vi "Do.vi"(8 "error in (no error)":errorcluster, 10 "Actor in":refnum<class "Actor.lvclass">, 11 "Concrete Tool Buttons Pressed Msg in":refnum<class "Concrete Tool Buttons Pressed Msg.lvclass">) -> (0 "error out":errorcluster, 2 "Actor out":refnum<class "Actor.lvclass">)   [LabVIEW 2020, in "Map View.lvlib" / "Concrete Tool Buttons Pressed Msg.lvclass"]
doc: "(<B>Filename</B>: Actor Framework.lvlib:Message.lvclass:Do.vi)\n\nDefines what a message does when it is received by an actor. Generally, a message instructs an actor to invoke one of its methods.\n\nBy default, this method does nothing. A child class must override it to define behavior. Create a child class by using the Actor Framework Message Maker dialog box."
uses:
  Concrete Tool Buttons Pressed Msg.lvclass
  E:/Project/Labview-Projects/Completed projects/Map Editor/Views/Tools View/Tools View Messages/Abstract Tool Buttons Pressed Msg/Abstract Tool Buttons Pressed Msg.lvclass
  <vilib>/ActorFramework/Actor/Actor.lvclass
  Map View/Map View.lvclass
  C:/Program Files/National Instruments/LabVIEW 2020/vi.lib/ActorFramework/Actor/Actor.lvclass
  Tools View/Tools View Messages/Abstract Tool Buttons Pressed Msg/Abstract Tool Buttons Pressed Msg.lvclass
panel:
  # "NOTICE -- YOU MUST LEAVE THIS NOTICE IN PLACE.\n\nCopyright (c) 2017, LIANG LIU Shawn.Liu.cn@gmail.com\nAll rights reserved.\n\nRedistribution and use in source and binary forms, with or without modification, are permitted provided that the following conditions are met:\n-Redistributions of source code must retain the above copyright notice, this list of conditions and the following disclaimer.\n-Redistributions in binary form must reproduce the above copyright notice, this list of conditions and the following disclaimer in the documentation and/or other materials provided with the distribution.\n-Neither the name of the eLp nor the names of its contributors may be used to endorse or promote products derived from this software without specific prior written permission.\n\nTHIS SOFTWARE IS PROVIDED BY THE COPYRIGHT HOLDERS AND CONTRIBUTORS \"AS IS\" AND ANY EXPRESS OR IMPLIED WARRANTIES, INCLUDING, BUT NOT LIMITED TO, THE IMPLIED WARRANTIES OF MERCHANTABILITY AND FITNESS FOR A PARTICULAR PURPOSE ARE DISCLAIMED. IN NO EVENT SHALL THE COPYRIGHT HOLDER OR CONTRIBUTORS BE LIABLE FOR ANY DIRECT, INDIRECT, INCIDENTAL, SPECIAL, EXEMPLARY, OR CONSEQUENTIAL DAMAGES (INCLUDING, BUT NOT LIMITED TO, PROCUREMENT OF SUBSTITUTE GOODS OR SERVICES; LOSS OF USE, DATA, OR PROFITS; OR BUSINESS INTERRUPTION) HOWEVER CAUSED AND ON ANY THEORY OF LIABILITY, WHETHER IN CONTRACT, STRICT LIABILITY, OR TORT (INCLUDING NEGLIGENCE OR OTHERWISE) ARISING IN ANY WAY OUT OF THE USE OF THIS SOFTWARE, EVEN IF ADVISED OF THE POSSIBILITY OF SUCH DAMAGE."
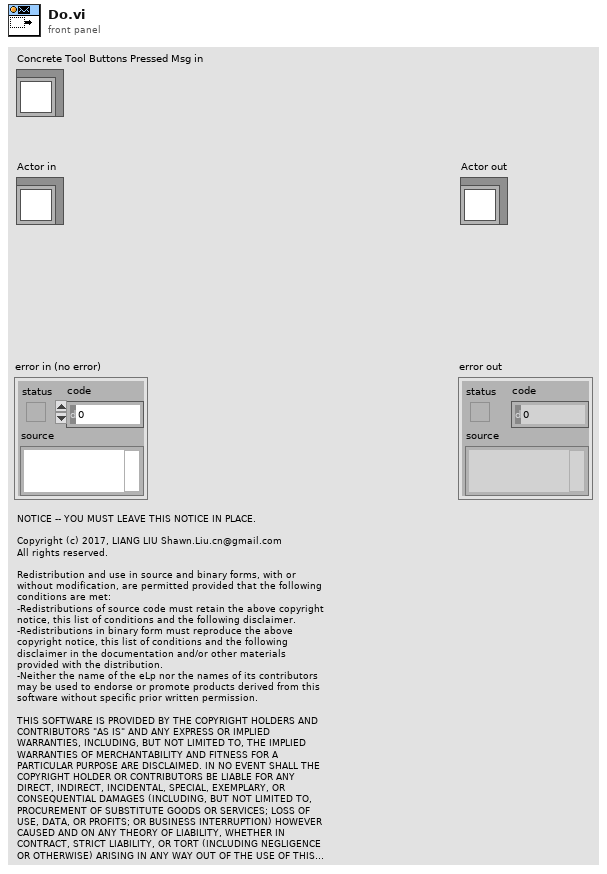
[diagram p1: front panel]
types:
  T1 = typedef "Tool Buttons.ctl" = enum32{"Pan Button", "Pencil Button", "Line Button", "Eraser Button", "Rectangle Select Button", "Deselect Button", "Crop Button", "Rotate Button", "Set Origin Button", "Zoom In Button", "Zoom Out Button"}
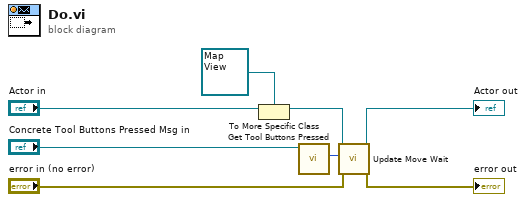
[diagram p0: block diagram]
diagram:
  n1 = To More Specific Class(target class=refnum<class "Map View.lvclass"> refnum ("Map View.lvlib:Map View.lvclass"), reference="Actor in") -> (specific class reference=w5:refnum<class "Map View.lvclass">)  [unwired: 1 in, 1 out]
  n2 = call "Get Tool Buttons Pressed.vi"("Abstract Tool Pressed Msg in"="Concrete Tool Buttons Pressed Msg in") -> ("Tool Buttons Pressed"=w1:T1)  [unwired: 9 in, 1 out]
  n3 = call "Update Move Wait.vi"("error in (no error)"="error in (no error)", "Tool Buttons"=w1, "Map View in"=w5) -> ("error out"=→"error out":errorcluster, "Map View out"=→"Actor out":refnum<class "Map View.lvclass">)  [unwired: 7 in]
